vi "Make Box on Graph.vi"(8 "Y2":dbl, 9 "Y1":dbl, 10 "X2":dbl, 11 "X1":dbl) -> (3 "Output Graph":cluster{dbl[], dbl[]})   [LabVIEW 2017]
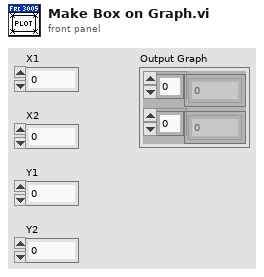
[diagram p1: front panel]
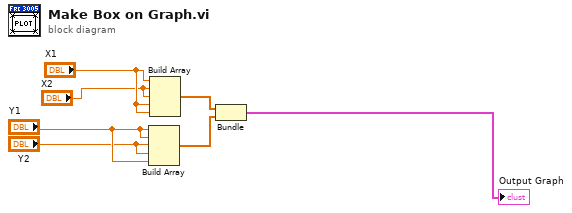
[diagram p0: block diagram]
diagram:
  n1 = Build Array("Y1", "Y1", "Y2", "Y2", "Y1") -> (w4:dbl[])
  n2 = Build Array("X1", "X2", "X2", "X1", "X1") -> (w3:dbl[])
  n3 = Bundle(w3, w4) -> (→"Output Graph":cluster{dbl[], dbl[]})  [unwired: 1 in]
